vi "Select Device.vi"(8 "error in (no error)":errorcluster, 10 "Selected":i32, 11 "Configuration Editor in":refnum<class "Configuration Editor.lvclass">) -> (0 "error out":errorcluster, 3 "Configuration Editor out":refnum<class "Configuration Editor.lvclass">)   [LabVIEW 2023, in "Configuration Editor.lvlib" / "Configuration Editor.lvclass"]
uses:
  Library/Configuration Editor.lvclass
  Library/Configuration Editor.lvclass/Configuration Editor.ctl
  builds/Framework/Configuration.lvlibp/Library/Configuration.lvclass
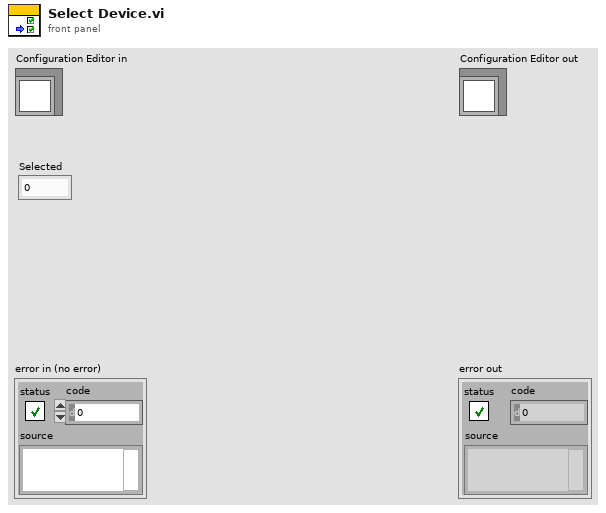
[diagram p1: front panel]
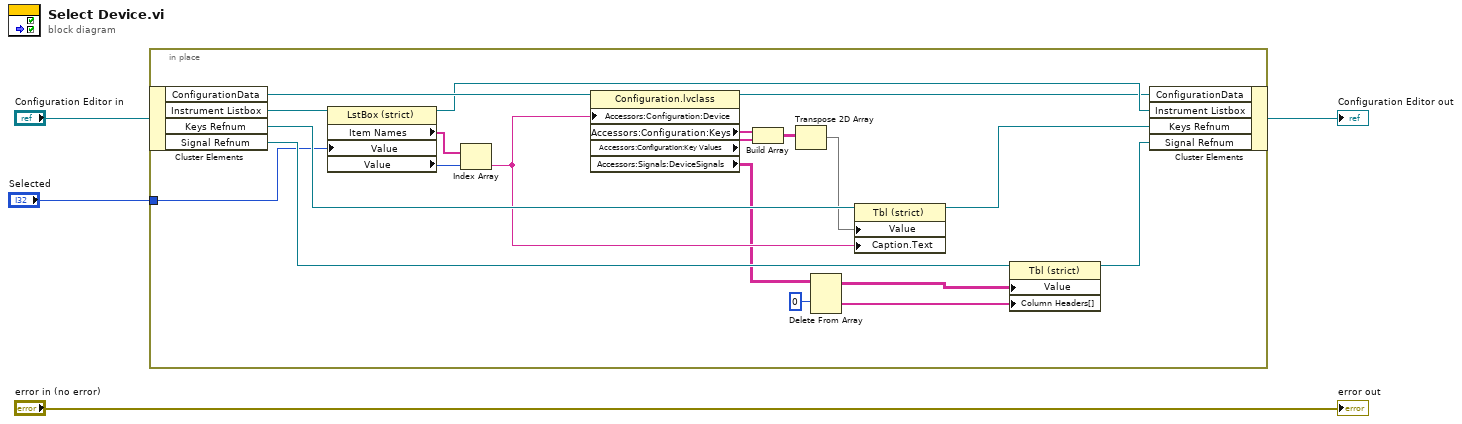
[diagram p0: block diagram]
diagram:
  n1 = in-place {
    in-place-border: "Selected" -> [w6]
    n2 = in-place-cluster #1("Configuration Editor in") -> ("ConfigurationData"=w24:refnum<class "Configuration.lvclass">, "Instrument Listbox"=w23:refnum<vi>, "Keys Refnum"=w19:refnum<vi>, "Signal Refnum"=w18:refnum<vi>)
    n3 = property class="LstBox (strict)"(reference=w23, "Value"=w6) -> (reference out=w21:refnum<vi>, "Item Names"=w22:string[], "Value"=w5:i32)  [unwired: 1 in, 1 out]
    n4 = Index Array(array=w22, index=w5) -> (element=w11:string)
    n5 = property class="Configuration.lvclass"(reference=w24, "Accessors:Configuration:Device"=w11) -> (reference out=w20:refnum<class "Configuration.lvclass">, "Accessors:Configuration:Keys"=w15:string[], "Accessors:Configuration:Key Values"=w14:string[], "Accessors:Signals:DeviceSignals"=w10:string[][])  [unwired: 1 in, 1 out]
    n6 = Build Array(w15, w14) -> (w13:string[][])
    n7 = Transpose 2D Array(2D array=w13) -> (transposed array=w12:string[][])
    n8 = Delete From Array(array=w10, index (row)=0) -> (deleted portion=w7:string[], array with subset deleted=w9:string[][])  [unwired: 2 in]
    n9 = property class="Tbl (strict)"(reference=w19, "Value"=w12, "Caption.Text"=w11) -> (reference out=w17:refnum<vi>)  [unwired: 1 in, 1 out]
    n10 = property class="Tbl (strict)"(reference=w18, "Value"=w9, "Column Headers[]"=w7) -> (reference out=w16:refnum<vi>)  [unwired: 1 in, 1 out]
    n11 = in-place-cluster #1("ConfigurationData"=w20, "Instrument Listbox"=w21, "Keys Refnum"=w17, "Signal Refnum"=w16) -> (→"Configuration Editor out":refnum<class "Configuration Editor.lvclass">)
  }
  "error out" <- "error in (no error)"
